vi "Force_Draft_Fan.vi"(8 "error in":errorcluster, 10 "NewVal":bool, 11 "Data":T1) -> (0 "error out":errorcluster, 3 "State":T2)   [LabVIEW 2023]
uses:
  Controls/State.ctl
  Controls/DataCluster.ctl
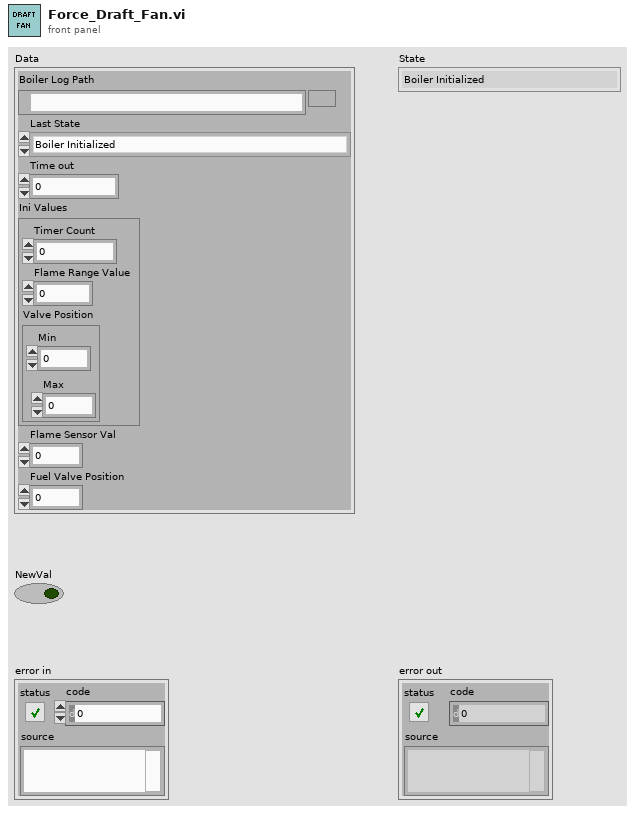
[diagram p1: front panel]
types:
  T1 = typedef "DataCluster.ctl" = cluster{"Boiler Log Path":path, "Last State":T2, "Time out":i32, "Ini Values":cluster{"Timer Count":dbl, "Flame Range Value":dbl, "Valve Position ":cluster{"Min":dbl, "Max":dbl}}, "Flame Sensor Val":dbl, "Fuel Valve Position":dbl}
  T2 = typedef "State.ctl" = enum16{"Boiler Initialized", "Boiler Ready", "Start Pre-Purge", "Pre-Purge Complete", "Pilot On", "Pilot Proved", "Force Draft Fan ON", "Boiler Running", "Start Shutdown Purge", "Shutdown Purge Complete", "Wait for Something"}
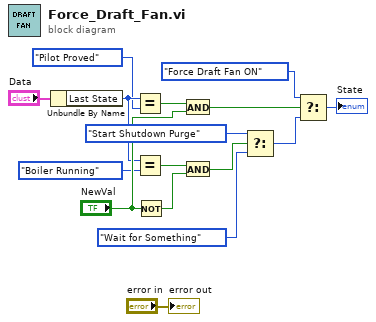
[diagram p0: block diagram]
diagram:
  n1 = Unbundle By Name("Data") -> ("Last State"=w7:T2)
  n2 = Equal?(x=w7, y=State."Pilot Proved") -> (x = y?=w4:bool)
  n3 = Equal?(x=w7, y=State."Boiler Running") -> (x = y?=w9:bool)
  n4 = Not(x="NewVal") -> (.not. x?=w10:bool)
  n5 = And(x=w4, y="NewVal") -> (x .and. y?=w11:bool)
  n6 = And(x=w9, y=w10) -> (x .and. y?=w13:bool)
  n7 = Select(t=State."Start Shutdown Purge" ("y"), s=w13, f=State."Wait for Something" ("y")) -> (s? t:f=w15:T2)
  n8 = Select(t=State."Force Draft Fan ON" ("y"), s=w11, f=w15) -> (s? t:f=→"State":T2)
  "error out" <- "error in"
